vi "popupwheel.vi"(6 "New Wheel Location":path, 9 "run number":string, 10 "runletter":string, 11 "Wheel Number":i16) -> (1 "run number out":string, 2 "runletter out":string, 3 "Wheel Number  out":string, 4 "New Wheel Location 2":path, 5 "Wheel Name":string)   [LabVIEW 2016]
doc: "loads wheel"
panel:
  in  "OK Button":bool
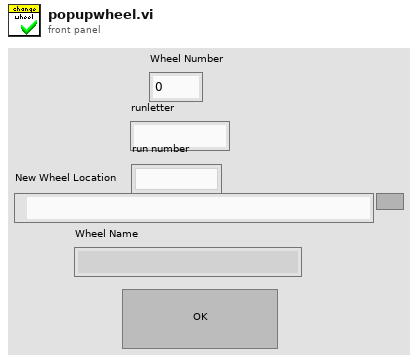
[diagram p1: front panel]
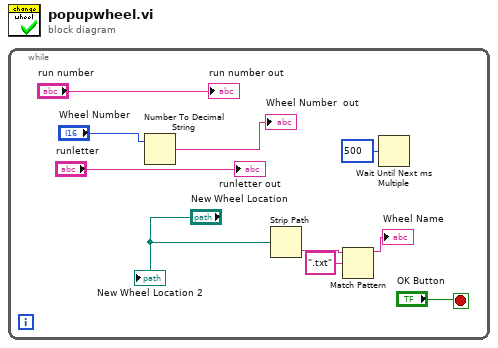
[diagram p0: block diagram]
diagram:
  n1 = while {
    stop <- "OK Button" stop-if-true
    n2 = Number To Decimal String(number="Wheel Number") -> (decimal integer string=→"Wheel Number  out":string)  [unwired: 1 in]
    n3 = Strip Path(path="New Wheel Location") -> (name=w6:string)  [unwired: 1 out]
    n4 = Match Pattern(string=w6, regular expression=".txt") -> (before substring=→"Wheel Name":string)  [unwired: 1 in, 3 out]
    n5 = Wait Until Next ms Multiple(millisecond multiple=u32 500) -> ()  [unwired: 1 out]
    "run number out" <- "run number"
    "runletter out" <- "runletter"
    "New Wheel Location 2" <- "New Wheel Location"
  }
